vi "SDSU_GetFrameTimeFromHardware.vi"(8 "error in":errorcluster, 10 "fd":i32, 11 "Database Ref":T1) -> (0 "errorout":errorcluster, 2 "frame_time":dbl, 4 "idle time":u32, 5 "total exp time":u32, 6 "min_exp_time":dbl)   [LabVIEW 2016]
uses:
  DBSHAND/private/vis/DatabaseHand_RefNum.ctl
  SDSU_GBLVariables.vi
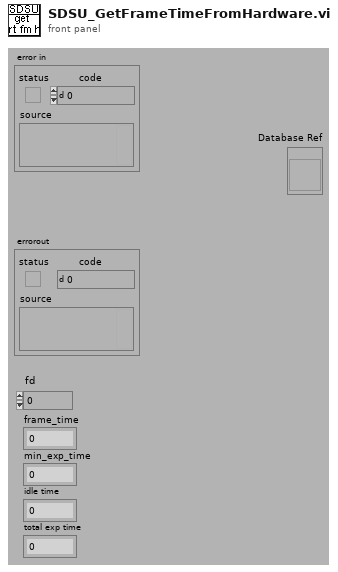
[diagram p1: front panel]
types:
  T1 = typedef "DatabaseHand_RefNum.ctl" = refnum<vi>
  T2 = typedef "CMN_TimingInfo.ctl" = cluster{"PixelTime":sgl, "SkipPixel":sgl, "SkipRow":sgl, "ShiftRow":sgl, "ShiftedPix":u16, "known_overhead":sgl, "DET_READ_TIME":sgl}
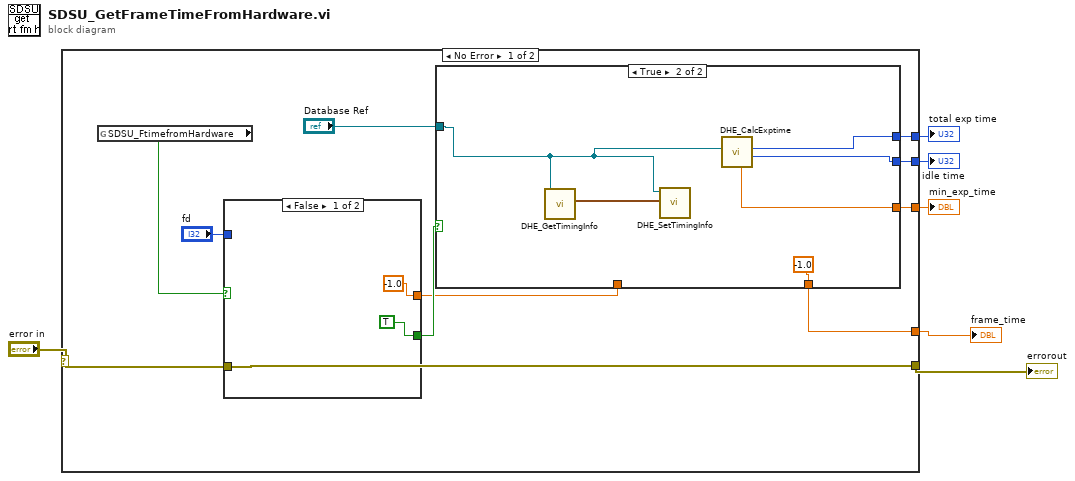
[diagram p0: block diagram]
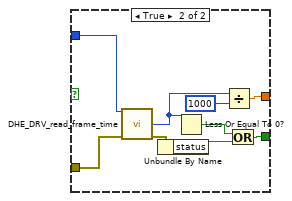
[diagram p2: hidden frame]
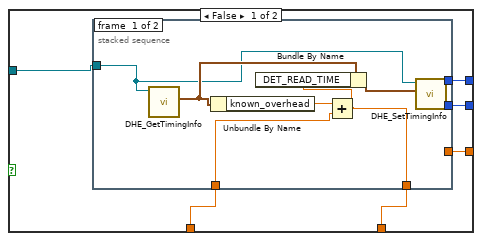
[diagram p3: hidden frame]
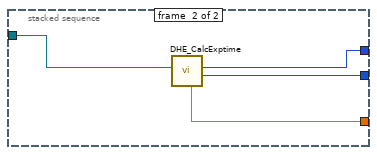
[diagram p4: hidden frame]
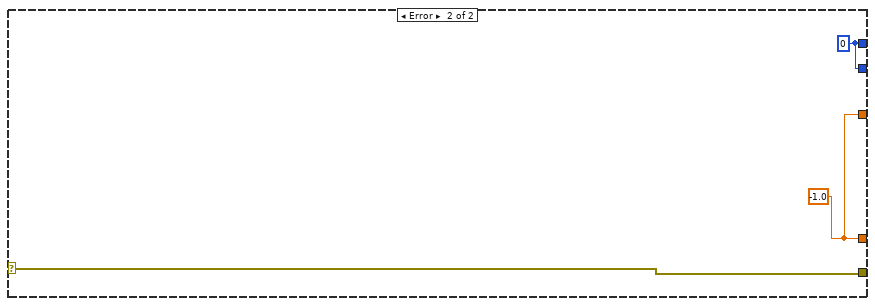
[diagram p5: hidden frame]
diagram:
  n1 = case shown="No Error" "error in" {
    selector: "error in" -> [w16 w52]
    tunnel: [w16 w52] -> w5
    tunnel: [w13 w51] -> w4
    tunnel: [w10 w51] -> w3
    tunnel: [w9 w50] -> w2
    tunnel: [w8 w50] -> w1
    frame No Error {
      n2 = global read "SDSU_GBLVariables.vi" "SDSU_FtimefromHardware"() -> (w11:bool)
      n3 = case shown="False" w11 {
        tunnel: w16 -> [_ w27]
        tunnel: "fd" -> [_ w21]
        tunnel: [TRUE w20] -> w14
        tunnel: [-1.0 w19] -> w12
        frame False {
        }
        frame True {
          n4 = call "DHE_DRV_read_frame_time.vi"("fd"=w21, "error in (no error)"=w27) -> ("return value"=w23:i32, "error out"=w26:errorcluster)  [unwired: 12 out]
          n5 = Unbundle By Name(w26) -> ("status"=w25:bool)
          n6 = Less Or Equal To 0?(x=w23) -> (x <= 0?=w24:bool)
          n7 = Divide(x=w23, y=1000) -> (x/y=w19:dbl)
          n8 = Or(x=w24, y=w25) -> (x .or. y?=w20:bool)
        }
      }
      n9 = case shown="True" w14 {
        tunnel: w12 -> [w33 _]
        tunnel: [w32 -1.0] -> w13
        tunnel: [w31 w47] -> w10
        tunnel: [w30 w48] -> w9
        tunnel: [w29 w49] -> w8
        tunnel: "Database Ref" -> [w28 w44]
        frame False {
          n10 = stacked-sequence {
            tunnel: w33 -> [w37 _]
            tunnel: [w36 _] -> w32
            tunnel: w28 -> [w34 w43]
            tunnel: [_ w42] -> w31
            tunnel: [_ w41] -> w30
            tunnel: [_ w40] -> w29
            frame #0 {
              n11 = call "DHE_GetTimingInfo.vi"("Database RefNum out"=w34) -> ("Timing"=w35:T2)  [unwired: 10 out]
              n12 = Unbundle By Name(w35) -> ("known_overhead"=w38:sgl)
              n13 = Add(x=w38, y=w37) -> (x+y=w36:dbl)
              n14 = Bundle By Name(cluster=w35, "DET_READ_TIME"=w36) -> (w39:T2)
              n15 = call "DHE_SetTimingInfo.vi"("Timing"=w39, "Database RefNum out"=w34) -> ()  [unwired: 10 out]
            }
            frame #1 {
              n16 = call "DHE_CalcExptime.vi"("DHE_DBSRef"=w43) -> ("idle time"=w41:u32, "total exp time"=w40:u32, "min_exp_time"=w42:dbl)  [unwired: 1 in, 7 out]
            }
          }
        }
        frame True {
          n17 = call "DHE_GetTimingInfo.vi"("Database RefNum out"=w44) -> ("Timing"=w45:T2)  [unwired: 10 out]
          n18 = call "DHE_SetTimingInfo.vi"("Timing"=w45, "Database RefNum out"=w44) -> ()  [unwired: 10 out]
          n19 = call "DHE_CalcExptime.vi"("DHE_DBSRef"=w44) -> ("idle time"=w48:u32, "total exp time"=w49:u32, "min_exp_time"=w47:dbl)  [unwired: 1 in, 7 out]
        }
      }
    }
    frame Error {
      w51 = -1.0
      w50 = u32 0 ("total exp time")
    }
  }
  "errorout" <- w5
  "frame_time" <- w4
  "min_exp_time" <- w3
  "idle time" <- w2
  "total exp time" <- w1
